vi "Convert State For Save 1.vi"(2 "Container State":T1, 3 "Display State":T2) -> (1 "Display State To Save":variant)   [LabVIEW 2013, in "XControl 1.xctl"]
uses:
  XControl 1.xctl
  State 1.ctl
  <vilib>/_xctls/Container State.ctl
  <vilib>/_xctls/XControlSupport.lvlib
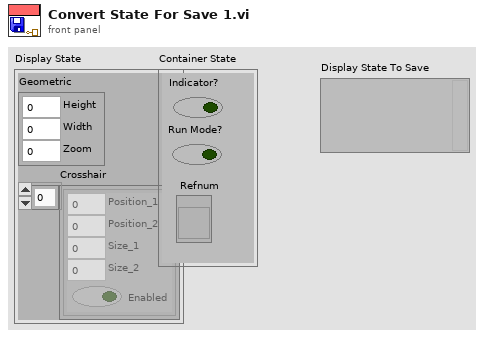
[diagram p1: front panel]
types:
  T1 = typedef "XControlSupport.lvlib/Container State.ctl" = cluster{"Indicator?":bool, "Run Mode?":bool, " Refnum":refnum<vi>}
  T2 = typedef "XControl 1.xctl/State 1.ctl" = cluster{"Geometric":cluster{"Height":dbl, "Width":dbl, "Zoom":dbl}, "Crosshair":cluster{"Position_1":dbl, "Position_2":dbl, "Size_1":dbl, "Size_2":dbl, "Enabled":bool}[]}
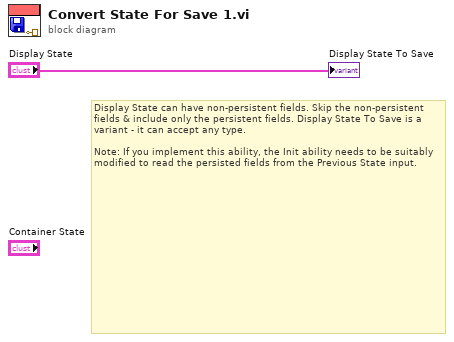
[diagram p0: block diagram]
diagram:
  # "Display State can have non-persistent fields. Skip the non-persistent fields & include only the persistent fields. Display State To Save is a variant - it can accept any type.\n\nNote: If you implement this ability, the Init ability needs to be suitably modified to read the persisted fields from the Previous State input."
  "Display State To Save" <- "Display State"
